vi "Tote Pusher (William).vi"(11 "Motor Output":dbl) -> (0 "Pusher Out":bool, 3 "Pusher In":bool)   [LabVIEW 2014]
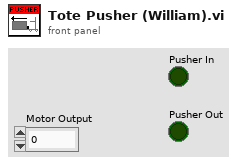
[diagram p1: front panel]
types:
  T1 = typedef "WPI_DigitalInputDevRef.ctl" = cluster{"DevStatus":errorcluster, "DIO Channel":T2, "Controller":T3}
  T2 = typedef "FPGA_DIOChannel.ctl" = enum8{"DIO 0", "DIO 1", "DIO 2", "DIO 3", "DIO 4", "DIO 5", "DIO 6", "DIO 7", "DIO 8", "DIO 9", "DIO MXP 0", "DIO MXP 1", "DIO MXP 2", "DIO MXP 3", "DIO MXP 4", "DIO MXP 5", "DIO MXP 6", "DIO MXP 7", "DIO MXP 8", "DIO MXP 9", "DIO MXP 10", "DIO MXP 11", "DIO MXP 12", "DIO MXP 13", "DIO MXP 14", "DIO MXP 15", "Invalid"}
  T3 = typedef "FPGA_TypedefDigitalModule.ctl" = enum16{"Controller 1"}
  T4 = typedef "WPI_MotorControlDeviceRef.ctl" = cluster{"DeviceStatus":errorcluster, "Type":T5, "PWM":cluster{"Controller":T3, "PWM Channel":T6, "DeadBand":T7}, "CAN":cluster{"Device Number":u8, "Control Mode":T8, "Semaphore":T9, "Max Vout":dbl, "TalonSRX Control Mode":T10}, "Invert":bool, "TransformRef":T11, "InvTransformRef":T11}
  T5 = typedef "WPI_MotorControlType.ctl" = enum16{"PWM", "CAN", "CANTalonSRX"}
  T6 = typedef "FPGA_DIOPWMChannel.ctl" = enum8{"PWM 0", "PWM 1", "PWM 2", "PWM 3", "PWM 4", "PWM 5", "PWM 6", "PWM 7", "PWM 8", "PWM 9", "PWM MXP 0", "PWM MXP 1", "PWM MXP 2", "PWM MXP 3", "PWM MXP 4", "PWM MXP 5", "PWM MXP 6", "PWM MXP 7", "PWM MXP 8", "PWM MXP 9", "Invalid"}
  T7 = typedef "WPI_PWMDeadband.ctl" = cluster{"Name":string, "maxPositivePwm":i32, "minPositivePwm":i32, "centerPwm":i32, "maxNegativePwm":i32, "minNegativePwm":i32, "angularRange":u16}
  T8 = typedef "WPI_CANJaguar_ControlMode.ctl" = enum8{"Percent VBus", "Current", "Speed", "Position", "Voltage"}
  T9 = typedef "Semaphore RefNum" = refnum<k1>
  T10 = typedef "WPI_CANTalonSRX_APIControlMode.ctl" = enum8{"Percent VBus", "Speed", "Position", "Slave", "Unchanged / Invalid"}
  T11 = typedef "WPI_PWMTransform_ConPane.ctl" = refnum<vi>
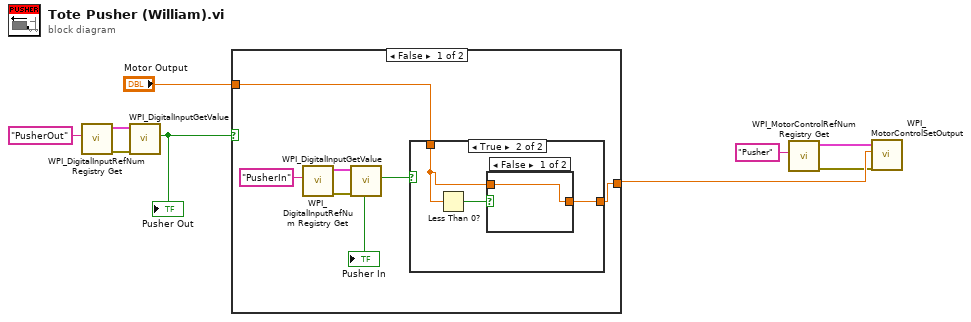
[diagram p0: block diagram]
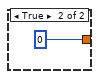
[diagram p3: hidden frame]
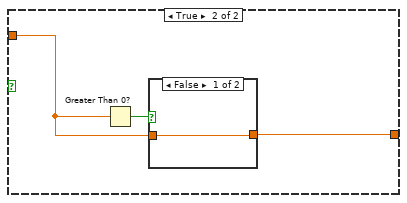
[diagram p4: hidden frame]
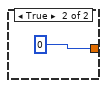
[diagram p5: hidden frame]
diagram:
  n1 = call <vilib>:"WPI_DigitalInputRefNum Registry Get.vi"("refnum name"="PusherOut") -> ("error out"=w4:errorcluster, "DigitalInputDevRef"=w3:T1)  [unwired: 9 in]
  n2 = call <vilib>:"WPI_DigitalInputGetValue.vi"("error in (no error)"=w4, "DigitalInputDevRef"=w3) -> ("Value"=w1:bool)  [unwired: 7 in, 2 out]
  "Pusher Out" <- w1
  n3 = case shown="False" w1 {
    tunnel: "Motor Output" -> [w15 w22]
    tunnel: [w14 w23] -> w8
    frame False {
      n4 = call <vilib>:"WPI_DigitalInputRefNum Registry Get.vi"("refnum name"="PusherIn") -> ("error out"=w13:errorcluster, "DigitalInputDevRef"=w12:T1)  [unwired: 9 in]
      n5 = call <vilib>:"WPI_DigitalInputGetValue.vi"("error in (no error)"=w13, "DigitalInputDevRef"=w12) -> ("Value"=w10:bool)  [unwired: 7 in, 2 out]
      "Pusher In" <- w10
      n6 = case shown="True" w10 {
        tunnel: w15 -> [w16 w17]
        tunnel: [w16 w18] -> w14
        frame False {
        }
        frame True {
          n7 = Less Than 0?(x=w17) -> (x < 0?=w19:bool)
          n8 = case shown="False" w19 {
            tunnel: [w20 0] -> w18
            tunnel: w17 -> [w20 _]
            frame False {
            }
            frame True {
            }
          }
        }
      }
    }
    frame True {
      n9 = Greater Than 0?(x=w22) -> (x > 0?=w24:bool)
      n10 = case shown="False" w24 {
        tunnel: [w25 0] -> w23
        tunnel: w22 -> [w25 _]
        frame False {
        }
        frame True {
        }
      }
    }
  }
  n11 = call <vilib>:"WPI_MotorControlRefNum Registry Get.vi"("refnum name"="Pusher") -> ("error out"=w5:errorcluster, "MotorControlDevRef"=w6:T4)  [unwired: 9 in]
  n12 = call <vilib>:"WPI_MotorControlSetOutput.vi"("error in (no error)"=w5, "Output"=w8, "MotorControlDevRef"=w6) -> ()  [unwired: 6 in, 3 out]
